vi "Exo3.vi"() -> ()   [LabVIEW 2019]
uses:
  <vilib>/Platform/TimedLoop/XDataNode/timing_clust.ctl
  <vilib>/Platform/TimedLoop/XDataNode/nitl_modes.ctl
  <vilib>/Platform/TimedLoop/XDataNode/wakeup.ctl
  <vilib>/myRIO/Instrument Drivers/Onboard Devices/Accelerometer/typedefs/Accelerometer Reference.ctl
  <vilib>/myRIO/Common/Instrument Driver Framework/Utilities/typedefs/myRIO Generic Hardware Reference.ctl
  <vilib>/myRIO/Common/Instrument Driver Framework/Utilities/typedefs/Hardware Version Enum.ctl
  <vilib>/myRIO/Common/Instrument Driver Framework/Utilities/typedefs/myRIO v1.0 Reference.ctl
  <vilib>/myRIO/Common/Instrument Driver Framework/Utilities/typedefs/Generic FPGA Reference.ctl
  <vilib>/myRIO/Common/Instrument Driver Framework/myRIO v1.0/Accelerometer/typedefs/Accelerometer Channels List.ctl
  <vilib>/myRIO/Common/Instrument Driver Framework/myRIO v1.0/Accelerometer/typedefs/Accelerometer Channels Enum.ctl
  <vilib>/userDefined/High Color/nirio_resource_hc.ctl
  <vilib>/myRIO/Instrument Drivers/Onboard IO/DIO/typedefs/DIO Reference.ctl
  <vilib>/myRIO/Common/Instrument Driver Framework/myRIO v1.0/DIO/typedefs/DIO Channels List.ctl
  <vilib>/myRIO/Common/Instrument Driver Framework/myRIO v1.0/DIO/typedefs/DIO Channels Enum.ctl
  <vilib>/myRIO/Common/Instrument Driver Framework/Utilities/vis/Is FPGA Ref Available.vi
  <vilib>/myRIO/Common/Instrument Driver Framework/myRIO v1.0/DIO/vis/myRIO v1.1 Open DIO.vi
  <vilib>/myRIO/Instrument Drivers/Onboard IO/DIO/vis/Read.vi
  <vilib>/myRIO/Common/Instrument Driver Framework/myRIO v1.0/Accelerometer/vis/myRIO v1.1 Open Accelerometer.vi
  <vilib>/myRIO/Instrument Drivers/Onboard Devices/Accelerometer/vis/Read.vi
  <vilib>/myRIO/Instrument Drivers/Onboard IO/DIO/vis/Write.vi
  <vilib>/myRIO/Common/Instrument Driver Framework/Utilities/vis/Validate Channels.vi
  <vilib>/myRIO/Common/Instrument Driver Framework/myRIO v1.0/DIO/vis/myRIO v1.0 Reserve DIO.vi
  <vilib>/myRIO/Common/Instrument Driver Framework/myRIO v1.0/Accelerometer/vis/myRIO v1.0 Reserve Accelerometer.vi
  <vilib>/myRIO/Common/Instrument Driver Framework/myRIO v1.0/Resource Manager/vis/myRIO v1.0 Reserve Channel List.vi
  <vilib>/myRIO/Common/Instrument Driver Framework/myRIO v1.0/DIO/vis/myRIO v1.0 Build MUX Configuration DIO.vi
  <vilib>/myRIO/Common/Instrument Driver Framework/myRIO v1.0/Accelerometer/vis/myRIO v1.0 Build MUX Configuration Accelerometer.vi
  <vilib>/myRIO/Common/Instrument Driver Framework/myRIO v1.0/Resource Manager/vis/myRIO v1.0 Reserve Channel.vi
  <vilib>/myRIO/Common/Instrument Driver Framework/myRIO v1.0/Resource Manager/vis/myRIO v1.0 Unreserve Channel.vi
  <vilib>/myRIO/Common/Instrument Driver Framework/myRIO v1.0/Resource Manager/vis/myRIO v1.0 Create Configuration List.vi
  <vilib>/myRIO/Common/Instrument Driver Framework/myRIO v1.0/Resource Manager/vis/myRIO v1.0 Build Mutex Name.vi
  <vilib>/Utility/VariantDataType/GetNumericInfo.vi
  <vilib>/Utility/error.llb/Error Cluster From Error Code.vi
  <vilib>/myRIO/Common/Instrument Driver Framework/myRIO v1.0/myRIO v1.1 Open.vi
  <vilib>/myRIO/Common/Instrument Driver Framework/myRIO v1.0/Accelerometer/vis/myRIO v1.0 Get Scaling Constant Accelerometer.vi
  <vilib>/myRIO/Common/Instrument Driver Framework/Utilities/vis/IO Manager.vi
  <vilib>/myRIO/Common/Instrument Driver Framework/Utilities/vis/Configuration Manager.vi
  <vilib>/myRIO/Common/Instrument Driver Framework/myRIO v1.0/myRIO v1.0 Close.vi
  <vilib>/myRIO/Common/Instrument Driver Framework/myRIO v1.0/Accelerometer/vis/myRIO v1.0 Read Accelerometer.vi
  <vilib>/myRIO/Common/Instrument Driver Framework/myRIO v1.0/Resource Manager/vis/myRIO v1.0 Configure IO.vi
  <vilib>/myRIO/Common/Instrument Driver Framework/myRIO v1.0/DIO/vis/myRIO v1.0 Read DIO.vi
  <vilib>/myRIO/Common/Instrument Driver Framework/myRIO v1.0/DIO/vis/myRIO v1.0 Write DIO.vi
  <vilib>/platform/TimedLoop/XDataNode/XDataNode.xnode
  <vilib>/myRIO/Express VI/Onboard Devices/Accelerometer/Accelerometer Express VI.xnode
  <vilib>/myRIO/Instrument Drivers/Onboard Devices/Accelerometer/vis/myRIO Accelerometer Open.xnode
  <vilib>/myRIO/Express VI/Onboard Devices/Button/Button Express VI.xnode
  <vilib>/myRIO/Instrument Drivers/Onboard IO/DIO/vis/myRIO DIO Open.xnode
  <vilib>/myRIO/Express VI/Onboard Devices/LED/LED Express VI.xnode
  <vilib>/myRIO/Instrument Drivers/Onboard Devices/Accelerometer/Accelerometer.lvlib
  <vilib>/myRIO/Instrument Drivers/Onboard IO/DIO/DIO.lvlib
  <vilib>/Platform/TimedLoop/XDataNode/XDNodeRunTimeDep.lvlib
panel:
  out "Numeric":dbl
  out "error IO 4":errorcluster
  out "Y3":dbl(graph)
  out "stop?":bool
  out "error IO 3":errorcluster
  in  "stop":bool
  out "error IO 2":errorcluster
  out "result 1":dbl(graph)
  out "diff":dbl(graph)
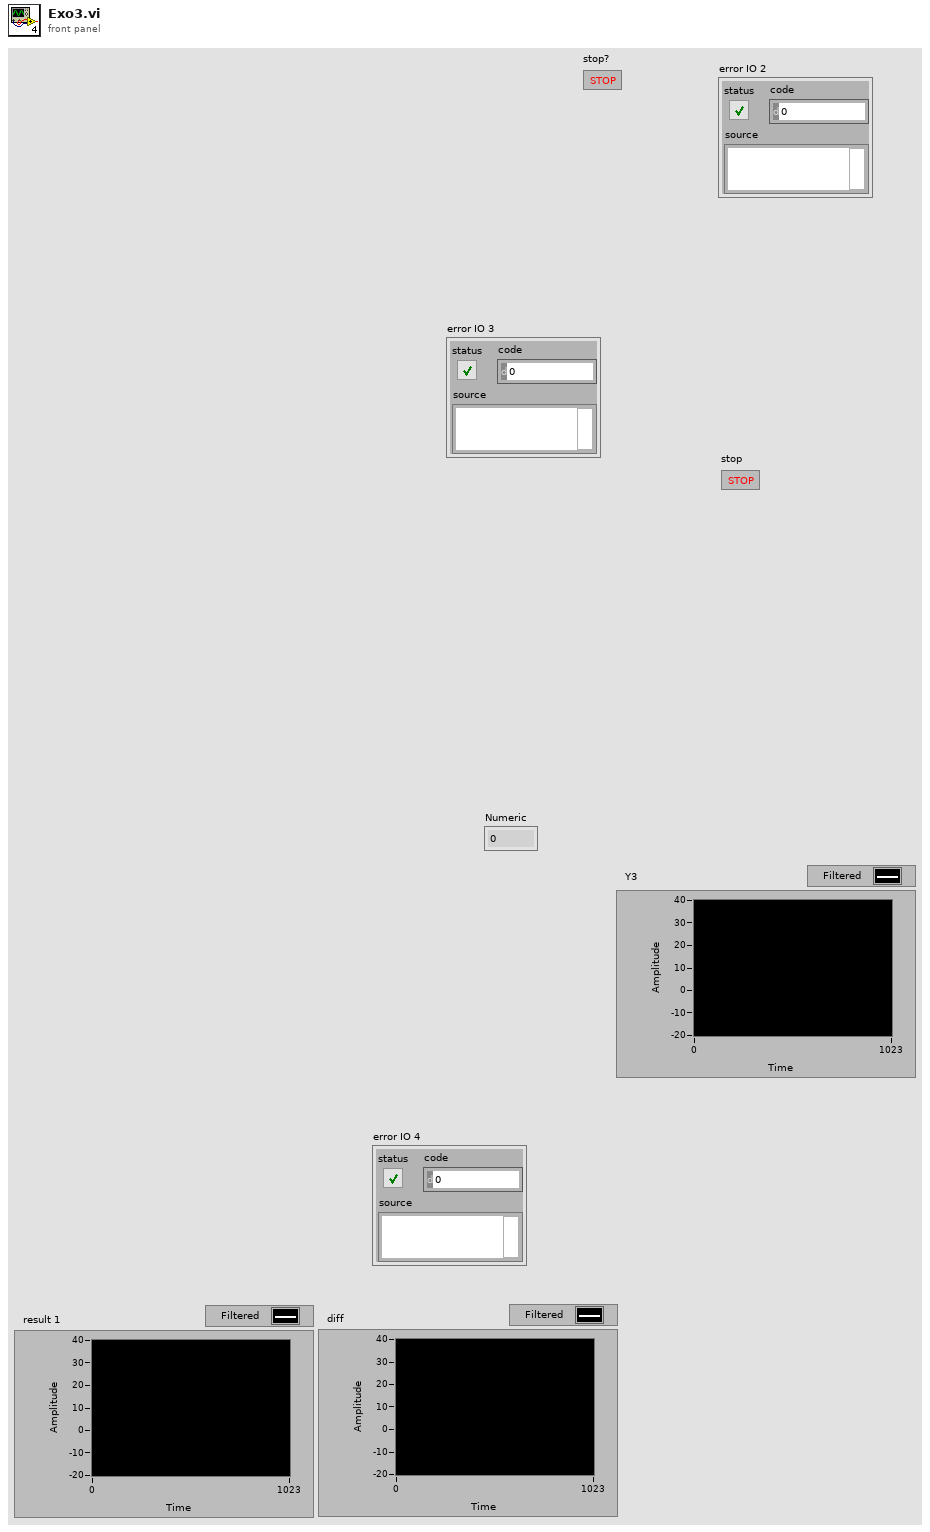
[diagram p1: front panel]
types:
  T1 = typedef "DIO.lvlib/DIO Reference.ctl" = cluster{"myRIO Reference":T2, "DIO Channels List":T6}
  T2 = typedef "myRIO Generic Hardware Reference.ctl" = cluster{"myRIO Model":T3, "myRIO Hardware Reference":T4}
  T3 = typedef "Hardware Version Enum.ctl" = enum16{"Unknown", "myRIO-1900", "myRIO-1950", "roboRIO", "NI ELVIS RIO CM", "ELVIS III"}
  T4 = typedef "myRIO v1.0 Reference.ctl" = cluster{"Generic FPGA Reference":T5, "Allow multiple opens":bool}
  T5 = typedef "Generic FPGA Reference.ctl" = refnum<k20>
  T6 = typedef "DIO Channels List.ctl" = T7[]
  T7 = typedef "DIO Channels Enum.ctl" = enum16{"Not Connected", "C/DIO0", "C/DIO1", "C/DIO2", "C/DIO3", "C/DIO4", "C/DIO5", "C/DIO6", "C/DIO7", "A/DIO0", "A/DIO1", "A/DIO2", "A/DIO3", "A/DIO4", "A/DIO5", "A/DIO6", "A/DIO7", "A/DIO8", "A/DIO9", "A/DIO10", "A/DIO11", "A/DIO12", "A/DIO13", "A/DIO14", "A/DIO15", "A/DIO16", "A/DIO17", "A/DIO18", "A/DIO19", "B/DIO0", "B/DIO1", "B/DIO2", "B/DIO3", "B/DIO4", "B/DIO5", "B/DIO6", "B/DIO7", "B/DIO8", "B/DIO9", "B/DIO10", "B/DIO11", "B/DIO12", "B/DIO13", "B/DIO14", "B/DIO15", "B/DIO16", "B/DIO17", "B/DIO18", "B/DIO19", "LED0", "LED1", "LED2", "LED3", "Button0", "DIO/DIO0", "DIO/DIO1", "DIO/DIO2", "DIO/DIO3", "DIO/DIO4", "DIO/DIO5", "DIO/DIO6", "DIO/DIO7", "DIO/DIO8", "DIO/DIO9", "SPI/CS0", "SPI/CS1", "SPI/CS2", "SPI/CS3", "LED RADIO (Green)", "LED RADIO (Red)", "LED COMM (Green)", "LED COMM (Red)", "LED MODE (Green)", "LED MODE (Red)"}
  T8 = typedef "nirio_resource_hc.ctl" = tag
  T9 = typedef "Accelerometer.lvlib/Accelerometer Reference.ctl" = cluster{"myRIO Reference":T2, "Accelerometer Channels List":T10, "LSB Weight":dbl}
  T10 = typedef "Accelerometer Channels List.ctl" = T11[]
  T11 = typedef "Accelerometer Channels Enum.ctl" = enum16{"Not Connected", "X-Axis", "Y-Axis", "Z-Axis"}
  T12 = typedef "XDNodeRunTimeDep.lvlib/timing_clust.ctl" = cluster{"Expected End [f-1]":u64, "Actual End [f-1]":u64, "Finished Late? [f-1]":bool, "Expected End [i-1]":u64, "Actual End [i-1]":u64, "Finished Late? [i-1]":bool, "Expected Start [i]":u64, "Actual Start [i]":u64, "Expected Start [f]":u64, "Actual Start [f]":u64, "Source Name":string, "Structure Name":string, "Period":i64, "Deadline":i64, "Offset":i64, "Start":i64, "Priority":i32, "Timeout":i32, "Mode":T13, "Wakeup Reason":T14, "Error":errorcluster, "Source Type":string, "Secondary Source Type":string, "Global End Time":u64, "Global Start Time":u64, "Frame Duration":u64, "Iteration Duration":u64, "Assigned CPU":i32, "I/O Scan Engine Mode":u32}
  T13 = typedef "XDNodeRunTimeDep.lvlib/nitl_modes.ctl" = enum32{"No Change", "Process missed periods, maintain original phase", "Discard missed periods, maintain original phase", "Process missed periods, ignore original phase", "Discard missed periods, ignore original phase"}
  T14 = typedef "XDNodeRunTimeDep.lvlib/wakeup.ctl" = enum32{"Normal", "Aborted", "Asynchronous wakeup", "Timing source error", "Timed loop error", "Timeout"}
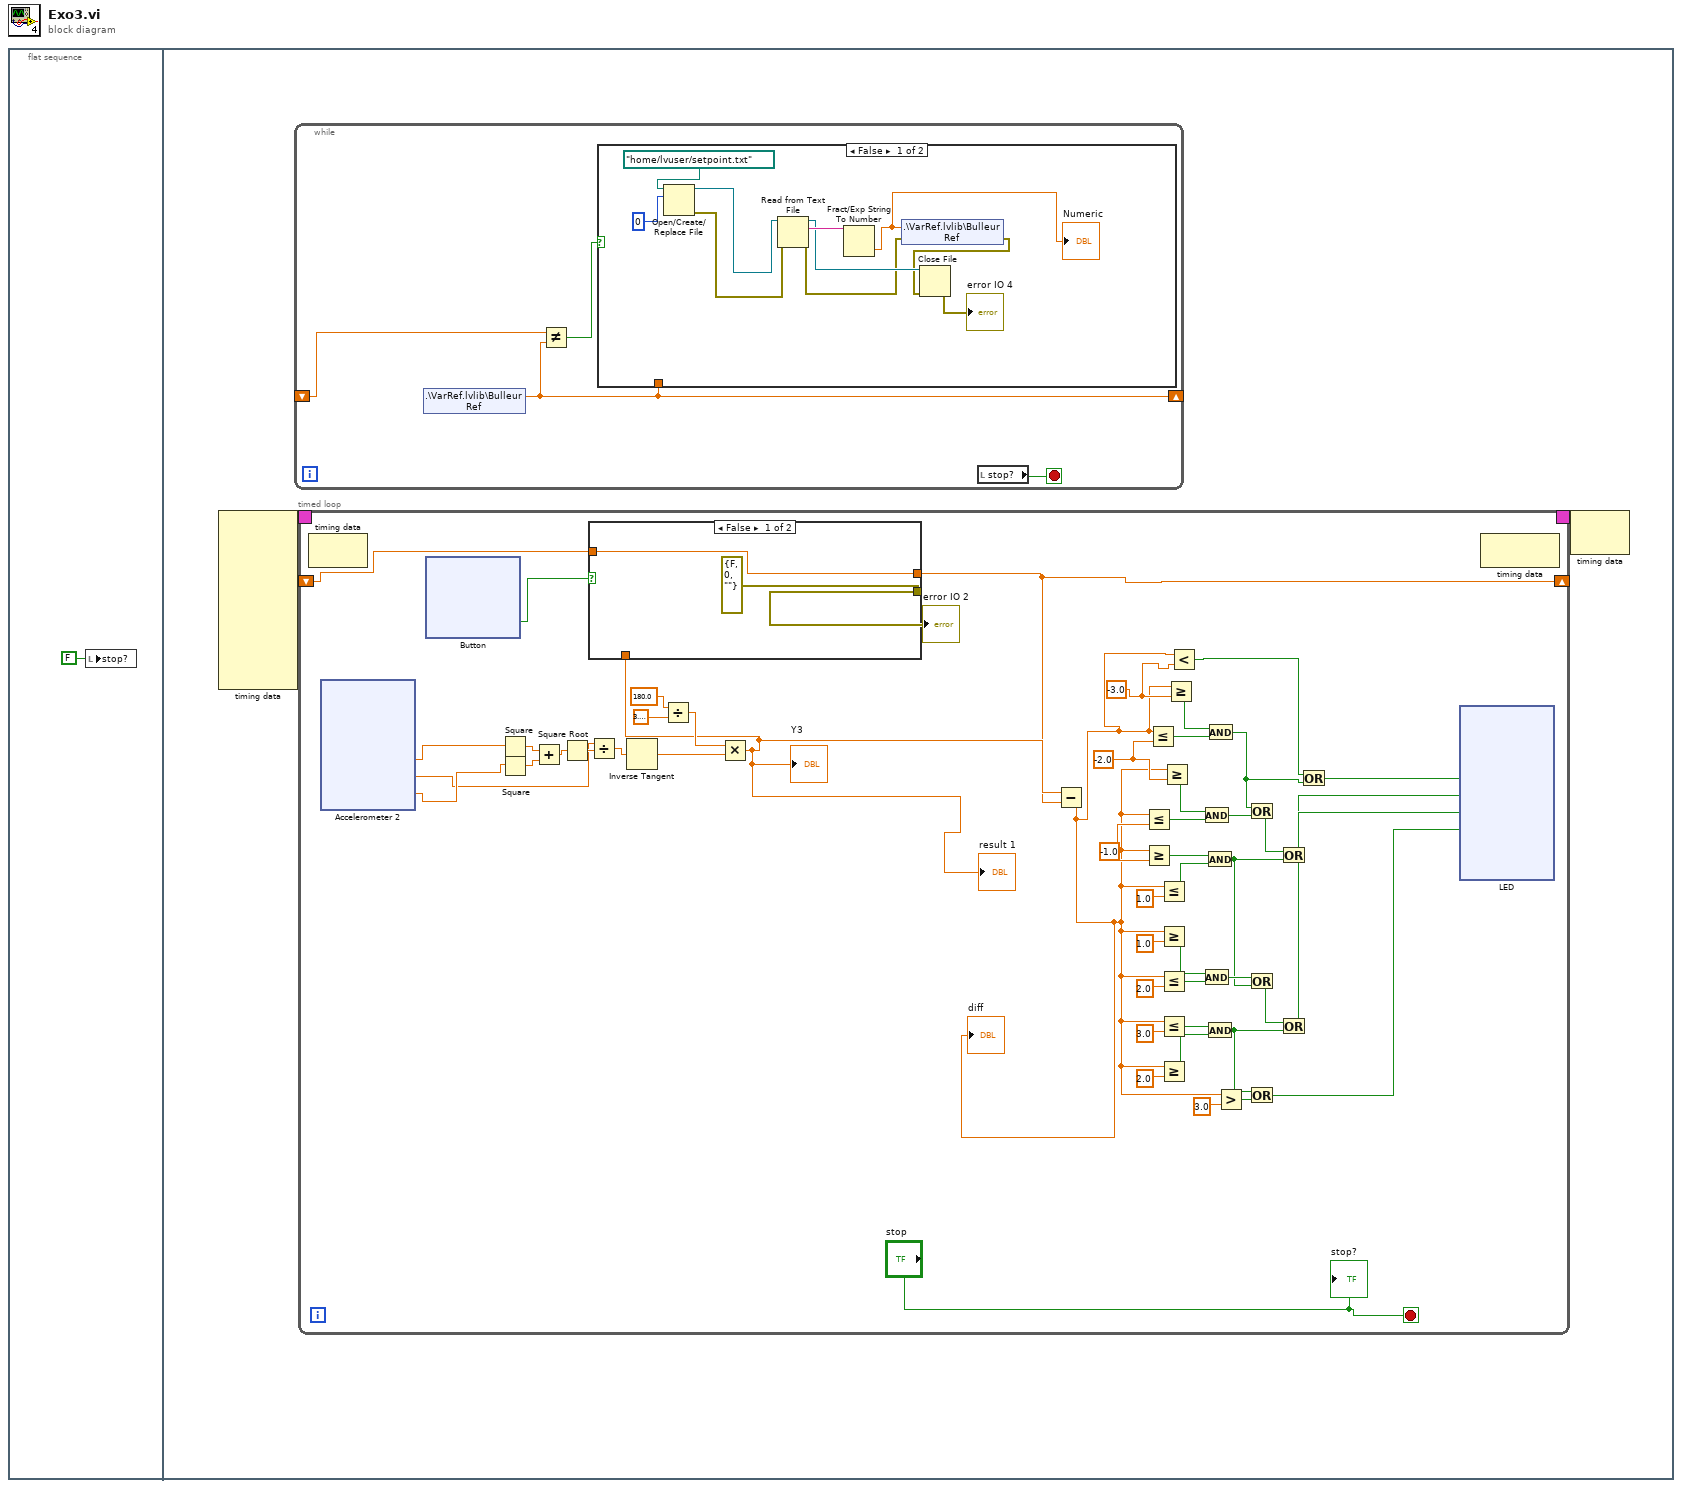
[diagram p0: block diagram]
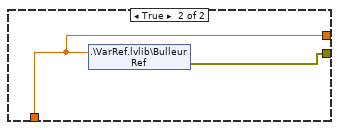
[diagram p2: hidden frame]
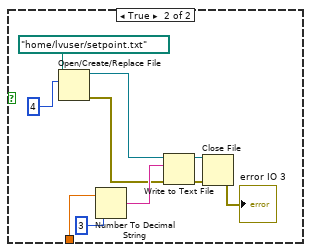
[diagram p3: hidden frame]
diagram:
  n1 = flat-sequence {
    frame #0 {
      n2 = local write "stop?"(FALSE ("stop?")) -> ()
    }
    frame #1 {
      n3 = node-c288() -> (w3:T12)  [unwired: 10 in]
      n4 = while {
        shift-right: [w176] -> _
        shift-left: _ -> [w178]
        stop <- w175 stop-if-true
        n5 = shared-variable ".\\VarRef.lvlib\\Bulleur Ref"() -> (w176:dbl)  [unwired: 1 in, 1 out]
        n6 = Not Equal?(x=w178, y=w176) -> (x != y?=w177:bool)
        n7 = case shown="False" w177 {
          tunnel: w176 -> [_ w197]
          frame False {
            n8 = Open/Create/Replace File(file path (use dialog)=path "/home/lvuser/setpoint.txt", operation (0:open)=0) -> (refnum out=w186:refnum<file>, error out=w185:errorcluster)  [unwired: 4 in, 1 out]
            n9 = Read from Text File(file (use dialog)=w186, error in=w185) -> (refnum out=w183:refnum<file>, text=w184:string, error out=w182:errorcluster)  [unwired: 2 in, 1 out]
            n10 = Fract/Exp String To Number(string=w184) -> (number=w180:dbl)  [unwired: 3 in, 1 out]
            "Numeric" <- w180
            n11 = shared-variable ".\\VarRef.lvlib\\Bulleur Ref"(w180, error in=w182) -> (error out=w181:errorcluster)
            n12 = Close File(refnum=w183, error in=w181) -> (error out=→"error IO 4":errorcluster)  [unwired: 1 out]
          }
          frame True {
            n13 = Open/Create/Replace File(file path (use dialog)=path "/home/lvuser/setpoint.txt", operation (0:open)=4) -> (refnum out=w195:refnum<file>, error out=w194:errorcluster)  [unwired: 4 in, 1 out]
            n14 = Number To Decimal String(number=w197, width (-)=3) -> (decimal integer string=w196:string)
            n15 = Write to Text File(file (use dialog)=w195, text=w196, error in=w194) -> (refnum out=w192:refnum<file>, error out=w191:errorcluster)  [unwired: 1 in, 1 out]
            n16 = Close File(refnum=w192, error in=w191) -> (error out=→"error IO 3":errorcluster)  [unwired: 1 out]
          }
        }
        n17 = local read "stop?"() -> (w175:bool)
      }
      n18 = timed-loop {
        timing: w3 -> [_]
        timing-out: [_] -> w2
        shift-right: [w37] -> _
        shift-left: _ -> [w52]
        stop <- "stop" stop-if-true
        w6 = -3.0
        w8 = -2.0
        w12 = -1.0
        n19 = node-c288() -> ()  [unwired: 1 in, 1 out]
        n20 = xnode "Accelerometer 2"() -> ("X-Axis"=w40:dbl, "Y-Axis"=w39:dbl, "Z-Axis"=w50:dbl)  [unwired: 1 in, 1 out]
        n21 = xnode "Button"() -> ("Value"=w54:bool)  [unwired: 1 in, 1 out]
        n22 = Square(x=w40) -> (x^2=w49:dbl)
        n23 = Square(x=w50) -> (x^2=w48:dbl)
        n24 = Add(x=w49, y=w48) -> (x+y=w47:dbl)
        n25 = Square Root(x=w47) -> (sqrt(x)=w46:dbl)
        n26 = Divide(x=w39, y=w46) -> (x/y=w45:dbl)
        n27 = Inverse Tangent(1:w45) -> (0:w41:dbl)
        n28 = Divide(x=180.0, y=3.141592653589793) -> (x/y=w42:dbl)
        n29 = Multiply(x=w42, y=w41) -> (x*y=w38:dbl)
        "result 1" <- w38
        "Y3" <- w38
        n30 = case shown="False" w54 {
          tunnel: w38 -> [_ w96]
          tunnel: [errorcluster {"status"=FALSE, "code"=0, "source"=""} ("error IO") w95] -> w53
          tunnel: [w93 w96] -> w37
          tunnel: w52 -> [w93 _]
          frame False {
          }
          frame True {
            n31 = shared-variable ".\\VarRef.lvlib\\Bulleur Ref"(w96) -> (error out=w95:errorcluster)  [unwired: 1 in]
          }
        }
        "error IO 2" <- w53
        n32 = Subtract(x=w38, y=w37) -> (x-y=w5:dbl)
        "diff" <- w5
        n33 = Less Or Equal?(x=w5, y=w12) -> (x <= y?=w13:bool)
        n34 = Greater Or Equal?(x=w5, y=w12) -> (x >= y?=w20:bool)
        n35 = Less Or Equal?(x=w5, y=w8) -> (x <= y?=w9:bool)
        n36 = Less Or Equal?(x=w5, y=1.0) -> (x <= y?=w19:bool)
        n37 = Greater Or Equal?(x=w5, y=1.0) -> (x >= y?=w24:bool)
        n38 = Less Or Equal?(x=w5, y=2.0) -> (x <= y?=w23:bool)
        n39 = Less Or Equal?(x=w5, y=3.0) -> (x <= y?=w31:bool)
        n40 = Greater Or Equal?(x=w5, y=2.0) -> (x >= y?=w30:bool)
        n41 = Greater Or Equal?(x=w5, y=w8) -> (x >= y?=w14:bool)
        n42 = Greater Or Equal?(x=w5, y=w6) -> (x >= y?=w10:bool)
        n43 = Less?(x=w5, y=w6) -> (x < y?=w4:bool)
        n44 = And(x=w14, y=w13) -> (x .and. y?=w11:bool)
        n45 = And(x=w24, y=w23) -> (x .and. y?=w22:bool)
        n46 = And(x=w20, y=w19) -> (x .and. y?=w15:bool)
        n47 = And(x=w31, y=w30) -> (x .and. y?=w28:bool)
        n48 = And(x=w10, y=w9) -> (x .and. y?=w7:bool)
        n49 = Greater?(x=w5, y=3.0) -> (0:w35:bool)
        n50 = Or(x=w7, y=w11) -> (x .or. y?=w18:bool)
        n51 = Or(x=w22, y=w15) -> (x .or. y?=w29:bool)
        n52 = Or(x=w28, y=w35) -> (x .or. y?=w34:bool)
        n53 = Or(x=w18, y=w15) -> (x .or. y?=w17:bool)
        n54 = Or(x=w29, y=w28) -> (x .or. y?=w27:bool)
        n55 = Or(x=w4, y=w7) -> (x .or. y?=w16:bool)
        n56 = xnode "LED"("LED0"=w16, "LED1"=w17, "LED2"=w27, "LED3"=w34) -> ()  [unwired: 1 in, 1 out]
        n57 = node-c288() -> ()  [unwired: 1 in, 1 out]
        "stop?" <- "stop"
      }
      n58 = node-c288(w2) -> ()  [unwired: 1 out]
    }
  }
